vi "template.vi"() -> ()   [LabVIEW 2014]
panel:
  out "modelName":string
  out "dim":i32
  out "initialPartition":i32[](array[numeric])
  out "data (1D)":dbl[](array[numeric])
  out "Error Message":string
  out "hcPair":dbl[][](array[numeric])
  out "Id":dbl
  out "m":i32
  out "II":dbl
  out "I":i32
  out "oneD":bool
  out "n":i32
  in  "minclus":i32=1
  in  "partition":i32[](array[numeric])
  in  "data":dbl[][](array[numeric])
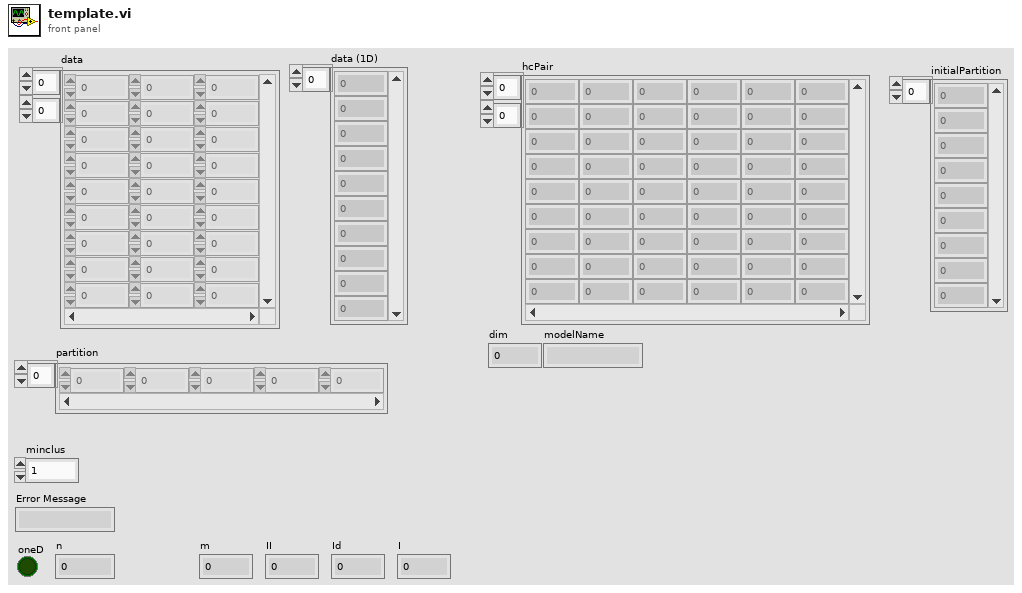
[diagram p1: front panel]
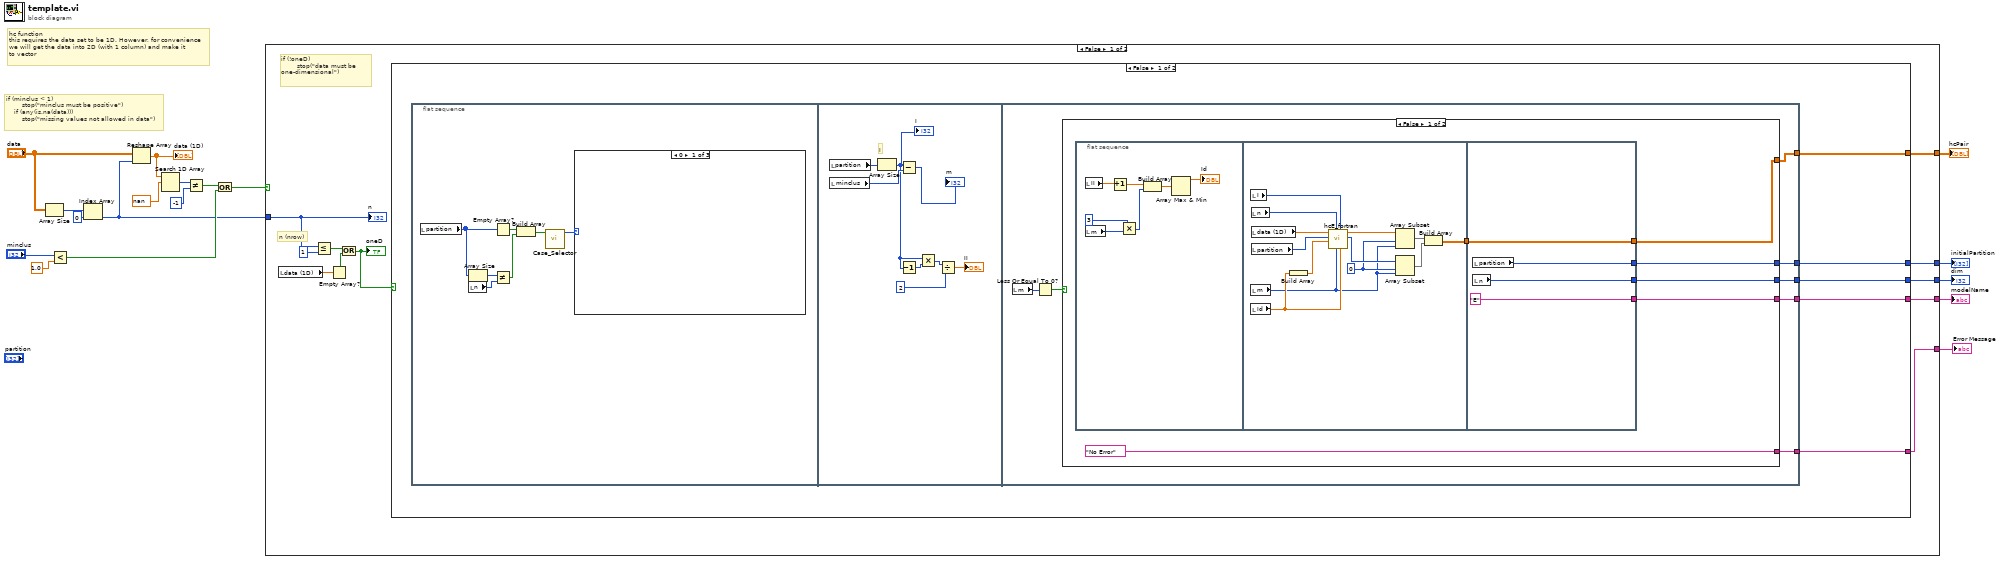
[diagram p0: block diagram]
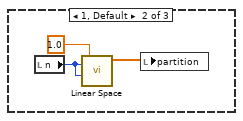
[diagram p2: hidden frame]
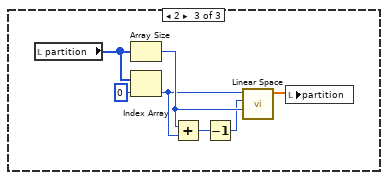
[diagram p3: hidden frame]
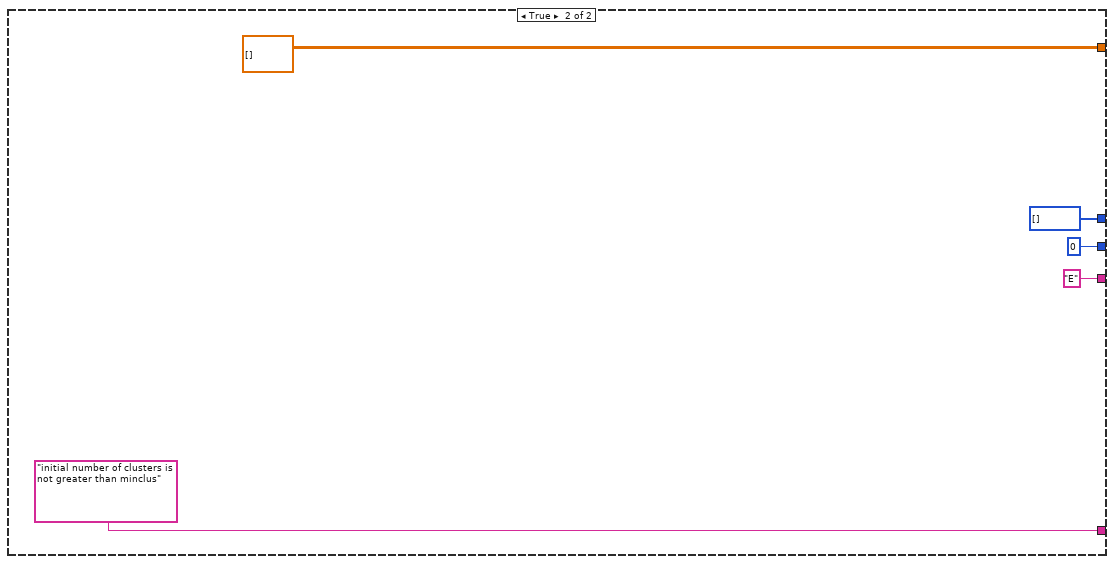
[diagram p4: hidden frame]
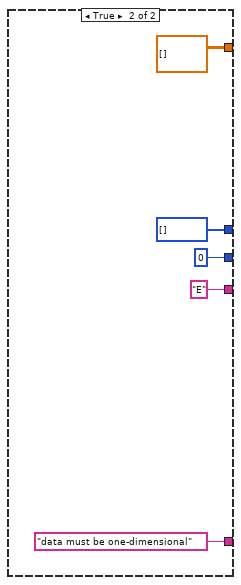
[diagram p5: hidden frame]
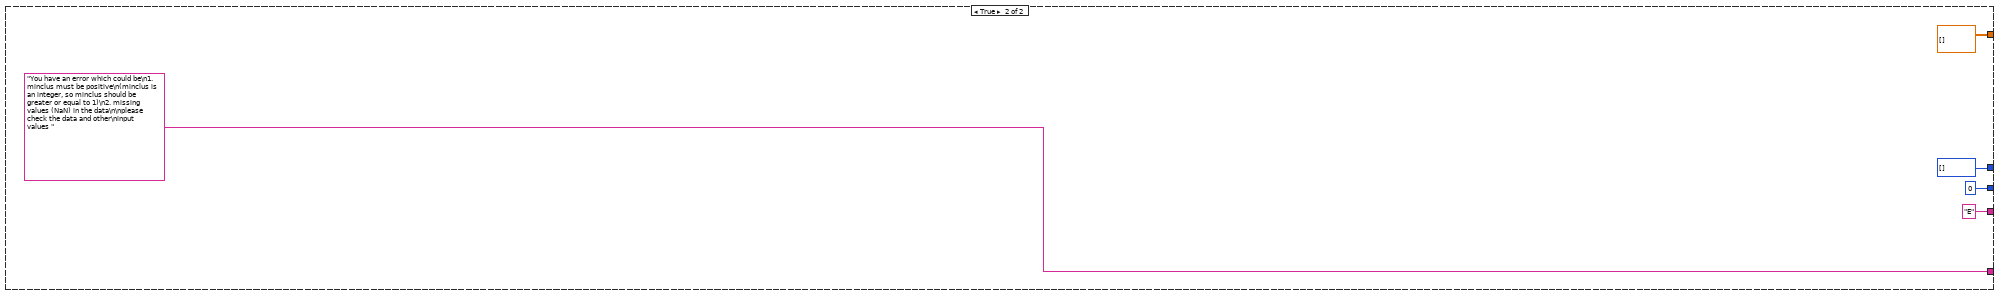
[diagram p6: hidden frame]
diagram:
  # "if (minclus < 1) \n        stop(\"minclus must be positive\")\n    if (any(is.na(data))) \n        stop(\"missing values not allowed in data\")"
  # "hc function\nthis requires the data set to be 1D. However, for convenience\nwe will get the data into 2D (with 1 column) and make it\nto vector"
  n1 = Array Size(array="data") -> (size(s)=w6:i32[])
  n2 = Less?(x="minclus", y=1.0) -> (x < y?=w11:bool)
  n3 = Index Array(array=w6, index=0) -> (element=w4:i32)
  n4 = Reshape Array("data", w4) -> (w16:dbl[])
  "data (1D)" <- w16
  n5 = Search 1D Array(1D array=w16, element=nan) -> (index of element=w14:i32)  [unwired: 1 in]
  n6 = Not Equal?(x=w14, y=-1) -> (x != y?=w12:bool)
  n7 = Or(x=w12, y=w11) -> (x .or. y?=w10:bool)
  n8 = case shown="False" w10 {
    tunnel: [w29 dbl[][] [] ("data")] -> w8
    tunnel: [w28 "You have an error which could be\n1. minclus must be positive\n(minclus is an integer, so minclus should be greater or equal to 1)\n2. missing values (NaN) in the data\n\nplease check the data and other\ninput values "] -> w7
    tunnel: w4 -> [w25 _]
    tunnel: [w21 i32[] [] ("partition")] -> w3
    tunnel: [w20 0 ("n")] -> w2
    tunnel: [w19 "E"] -> w1
    frame False {
      # "n (nrow)"
      # "if (!oneD) \n        stop(\"data must be one-dimensional\")"
      n9 = local read "data (1D)"() -> (w23:dbl[])
      n10 = Less Or Equal?(x=w25, y=1) -> (x <= y?=w27:bool)
      n11 = Empty Array?(array=w23) -> (empty?=w24:bool)
      n12 = Or(x=w27, y=w24) -> (x .or. y?=w22:bool)
      "oneD" <- w22
      n13 = case shown="False" w22 {
        tunnel: [w34 dbl[][] [] ("data")] -> w29
        tunnel: [w33 "data must be one-dimensional"] -> w28
        tunnel: [w32 i32[] [] ("partition")] -> w21
        tunnel: [w31 0 ("n")] -> w20
        tunnel: [w30 "E"] -> w19
        frame False {
          n14 = flat-sequence {
            tunnel: [w64] -> w34
            tunnel: [w63] -> w33
            tunnel: [w62] -> w32
            tunnel: [w61] -> w31
            tunnel: [w60] -> w30
            frame #0 {
              n15 = local read "partition"() -> (w41:i32[])
              n16 = Array Size(array=w41) -> (size(s)=w39:i32)
              n17 = local read "n"() -> (w40:i32)
              n18 = Empty Array?(array=w41) -> (empty?=w38:bool)
              n19 = Not Equal?(x=w39, y=w40) -> (x != y?=w37:bool)
              n20 = Build Array(w38, w37) -> (w36:bool[])
              n21 = call "Case_Selector.vi"("Array"=w36) -> ("Case Numer"=w35:i32)  [unwired: 10 in]
              n22 = case shown="0" w35 {
                frame 0 {
                }
                frame 1, Default {
                  n23 = local read "n"() -> (w42:i32)
                  n24 = call "Linear Space.vi"("Number of Samples"=w42, "Maximum"=w42, "Minimum"=1.0) -> ("Array"=w44:dbl[])  [unwired: 3 in, 1 out]
                  n25 = local write "partition"(w44) -> ()
                }
                frame 2 {
                  n26 = local read "partition"() -> (w49:i32[])
                  n27 = Array Size(array=w49) -> (size(s)=w48:i32)
                  n28 = Index Array(array=w49, index=0) -> (element=w47:i32)
                  n29 = Add(x=w48, y=w47) -> (x+y=w46:i32)
                  n30 = Decrement(x=w46) -> (x-1=w45:i32)
                  n31 = call "Linear Space.vi"("Number of Samples"=w48, "Maximum"=w45, "Minimum"=w47) -> ("Array"=w51:dbl[])  [unwired: 3 in, 1 out]
                  n32 = local write "partition"(w51) -> ()
                }
              }
            }
            frame #1 {
              # "I"
              n33 = local read "partition"() -> (w59:i32[])
              n34 = local read "minclus"() -> (w58:i32)
              n35 = Array Size(array=w59) -> (size(s)=w55:i32)
              "I" <- w55
              n36 = Subtract(x=w55, y=w58) -> (x-y=→"m":i32)
              n37 = Decrement(x=w55) -> (x-1=w56:i32)
              n38 = Multiply(x=w55, y=w56) -> (x*y=w54:i32)
              n39 = Divide(x=w54, y=2) -> (x/y=→"II":dbl)
            }
            frame #2 {
              n40 = local read "m"() -> (w66:i32)
              n41 = Less Or Equal To 0?(x=w66) -> (x <= 0?=w65:bool)
              n42 = case shown="False" w65 {
                tunnel: [w71 dbl[][] [] ("data")] -> w64
                tunnel: ["No Error" "initial number of clusters is not greater than minclus"] -> w63
                tunnel: [w69 i32[] [] ("partition")] -> w62
                tunnel: [w68 0 ("n")] -> w61
                tunnel: [w67 "E"] -> w60
                frame False {
                  n43 = flat-sequence {
                    tunnel: [w80] -> w70
                    tunnel: [w96] -> w71
                    tunnel: w70 -> [w96]
                    tunnel: [w95] -> w69
                    tunnel: [w94] -> w68
                    tunnel: ["E"] -> w67
                    frame #0 {
                      n44 = local read "II"() -> (w78:dbl)
                      n45 = local read "m"() -> (w77:i32)
                      n46 = Increment(x=w78) -> (x+1=w79:dbl)
                      n47 = Multiply(x=3, y=w77) -> (x*y=w73:i32)
                      n48 = Build Array(w79, w73) -> (w75:dbl[])
                      n49 = Array Max & Min(array=w75) -> (max value=→"Id":dbl)  [unwired: 3 out]
                    }
                    frame #1 {
                      w84 = 0
                      n50 = local read "I"() -> (w89:i32)
                      n51 = local read "m"() -> (w83:i32)
                      n52 = local read "Id"() -> (w88:dbl)
                      n53 = local read "n"() -> (w91:i32)
                      n54 = local read "data (1D)"() -> (w92:dbl[])
                      n55 = local read "partition"() -> (w90:i32[])
                      n56 = Build Array(w88) -> (w87:dbl[])
                      n57 = call "hcE_fortran.vi"("nd"=w88, "ng"=w89, "ns"=w83, "n"=w91, "d"=w87, "ic"=w90, "x (data)"=w92) -> ("ic (out)"=w85:i32[], "x (data out)"=w86:dbl[])  [unwired: 2 in, 1 out]
                      n58 = Array Subset(array=w86, index=w84, length=w83) -> (w82:dbl[])
                      n59 = Array Subset(array=w85, index=w84, length=w83) -> (w81:i32[])
                      n60 = Build Array(w82, w81) -> (w80:dbl[][])
                    }
                    frame #2 {
                      n61 = local read "partition"() -> (w95:i32[])
                      n62 = local read "n"() -> (w94:i32)
                    }
                  }
                }
                frame True {
                }
              }
            }
          }
        }
        frame True {
        }
      }
      "n" <- w25
    }
    frame True {
    }
  }
  "hcPair" <- w8
  "Error Message" <- w7
  "initialPartition" <- w3
  "dim" <- w2
  "modelName" <- w1
